vi "New Timed Average Buffer.vi"(8 "error in (no error)":errorcluster, 10 "Buffer Duration [s]":dbl=1.0, 11 "TimedBuffer in":refnum<class "TimedAverageBuffer.lvclass">) -> (0 "error out":errorcluster, 3 "Timed Average Buffer":T1)   [LabVIEW 2015, in "TimedAverageBuffer.lvlib" / "TimedAverageBuffer.lvclass"]
uses:
  TimedAverageBuffer.lvclass
  TimedAverageBuffer Reference.ctl
  TimedAverageBuffer.lvclass/TimedAverageBuffer.ctl
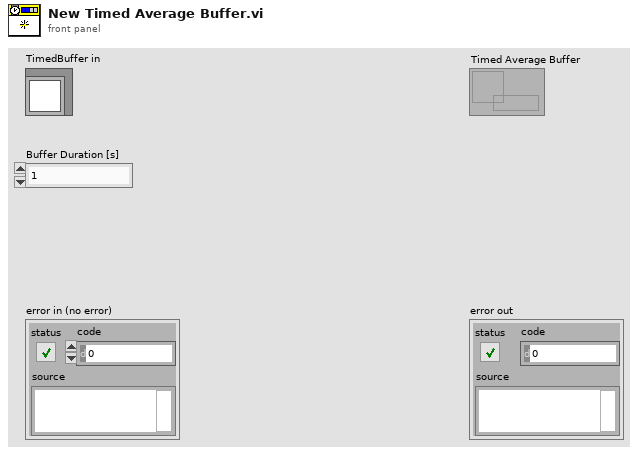
[diagram p1: front panel]
types:
  T1 = typedef "TimedAverageBuffer.lvlib/TimedAverageBuffer.lvclass/TimedAverageBuffer Reference.ctl" = refnum<data-value>
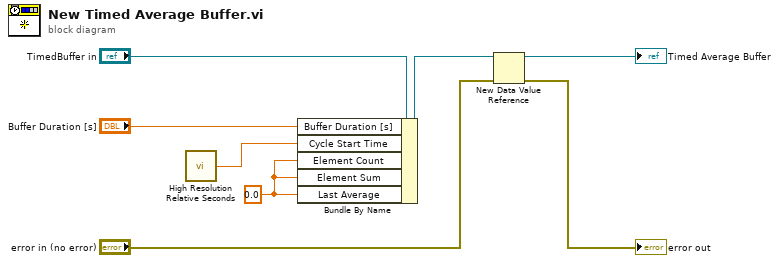
[diagram p0: block diagram]
diagram:
  w4 = 0.0 ("Last Average")
  n1 = call <vilib>:"High Resolution Relative Seconds.vi"() -> ("relative seconds"=w3:dbl)
  n2 = Bundle By Name(cluster="TimedBuffer in", "Buffer Duration [s]"="Buffer Duration [s]", "Cycle Start Time"=w3, "Element Count"=w4, "Element Sum"=w4, "Last Average"=w4) -> (w7:refnum<class "TimedAverageBuffer.lvclass">)
  n3 = New Data Value Reference(data value=w7, error in="error in (no error)") -> (data value reference=→"Timed Average Buffer":refnum<data-value>, error out=→"error out":errorcluster)
